vi "Get Result.vi"(4 "Controller name":string, 6 "Last request":bool, 8 "error in (no error)":errorcluster, 11 "Worker in":refnum<class "Worker Actor.lvclass">) -> (0 "error out":errorcluster, 2 "Result":refnum<class "Acquired Result.lvclass">, 3 "Worker out":refnum<class "Worker Actor.lvclass">)   [LabVIEW 2021, in "Worker Actor.lvclass"]
uses:
  Worker Actor.lvclass
  NHMFL_Core/Libraries/Instruments/Results/Acquired Result/Acquired Result.lvclass
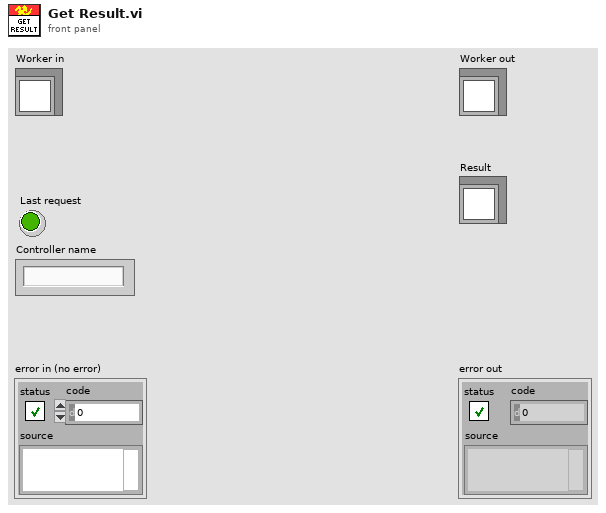
[diagram p1: front panel]
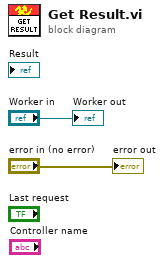
[diagram p0: block diagram]
diagram:
  "error out" <- "error in (no error)"
  "Worker out" <- "Worker in"
